vi "ReportControl.vi"(1 "Destination":T2={"Subsystem Id"=90, "Node Id"=1, "Component Id"=1}, 2 "Controller":T1={"ID"={"Subsystem Id"=90, "Node Id"=1, "Component Id"=1}, "Authority Code"=0}, 3 "Source":T2={"Subsystem Id"=3, "Node Id"=1, "Component Id"=1}) -> (0 "Encoded JAUS Message":string)   [LabVIEW 2009]
uses:
  Support Files/Address.ctl
  Support Files/JAUS Controller.ctl
panel:
  in  "Command Code":string="@\r"
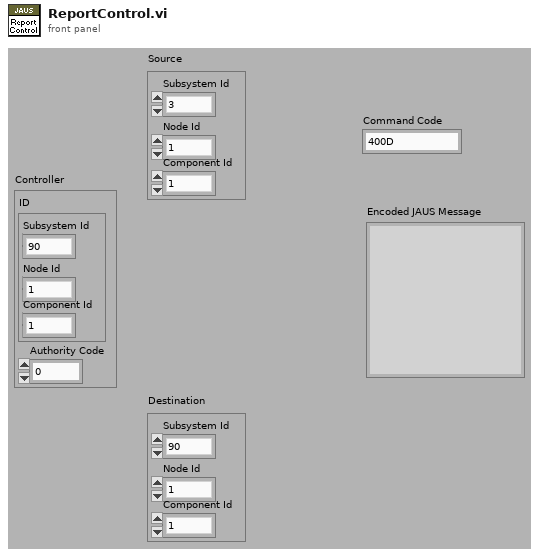
[diagram p1: front panel]
types:
  T1 = typedef "JAUS Controller.ctl" = cluster{"ID":T2, "Authority Code":u8}
  T2 = typedef "Address.ctl" = cluster{"Subsystem Id":u16, "Node Id":u8, "Component Id":u8}
  T3 = cluster{"unsigned byte array[0]":u8, "unsigned byte array[1]":u8}
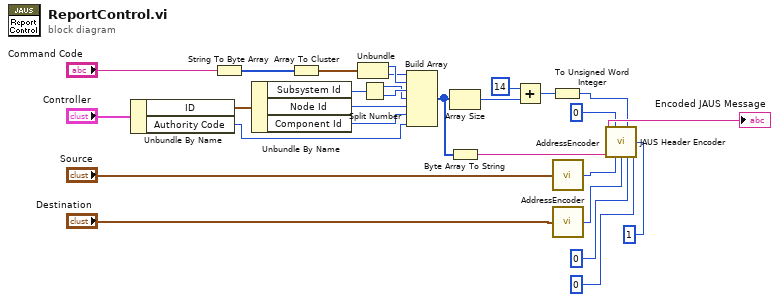
[diagram p0: block diagram]
diagram:
  n1 = Unbundle By Name("Controller") -> ("ID"=w2:T2, "Authority Code"=w1:u8)
  n2 = String To Byte Array(string="Command Code") -> (unsigned byte array=w15:u8[])
  n3 = Unbundle By Name(w2) -> ("Subsystem Id"=w11:u16, "Node Id"=w8:u8, "Component Id"=w7:u8)
  n4 = Array To Cluster(array=w15) -> (cluster=w14:T3)
  n5 = Unbundle(w14) -> ("unsigned byte array[0]"=w13:u8, "unsigned byte array[1]"=w12:u8)
  n6 = Split Number(x=w11) -> (hi(x)=w9:u8, lo(x)=w10:u8)
  n7 = Build Array(w12, w13, w10, w9, w8, w7, w1) -> (w19:u8[])
  n8 = Array Size(array=w19) -> (size(s)=w17:i32)
  n9 = Byte Array To String(unsigned byte array=w19) -> (string=w21:string)
  n10 = Add(x=14, y=w17) -> (x+y=w16:i32)
  n11 = To Unsigned Word Integer(number=w16) -> (unsigned 16bit integer=w4:u16)
  n12 = call "AddressEncoder.vi"("Address Cluster"="Source") -> ("Address"=w27:u32)
  n13 = call "AddressEncoder.vi"("Address Cluster"="Destination") -> ("Address"=w26:u32)
  n14 = call "JAUS Header Encoder.vi"("Message Type (0-5)"=u8 0, "Data Size (8-23)"=w4, "Priority(40-41)"=u8 1, "Payload"=w21, "Source ID (80-95)"=w27, "Destination ID (48-79)"=w26, "Data Flags (46-47)"=u8 0, "Ack/Nak (44-45)"=u8 0) -> ("Encoded JAUS Message"=→"Encoded JAUS Message":string)  [unwired: 7 in]
